vi "Part 2.vi"(11 "Input":string) -> (3 "Output":i64)   [LabVIEW 2021]
uses:
  d8bb4194-d316-453b-bd2f-f561d20e04f1.vi
  <userlib>/_OpenG.lib/string/string.llb/Convert EOLs (String)__ogtk.vi
  <vilib>/Comparison/Less/Less Functor/Less Functor.lvclass
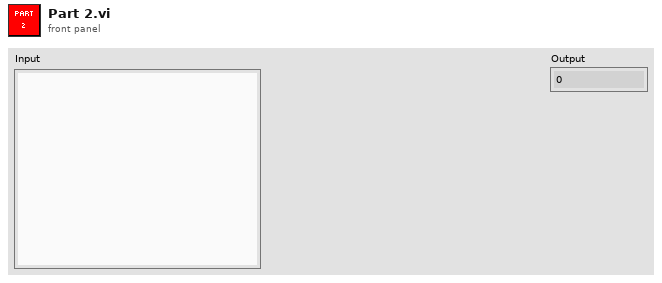
[diagram p1: front panel]
types:
  T1 = cluster{"Type":enum16{"High card", "One pair", "Two pair", "Three of a kind", "Full house", "Four of a kind", "Five of a kind"}, "Hand":string, "Bid":i64}
  T2 = enum16{"High card", "One pair", "Two pair", "Three of a kind", "Full house", "Four of a kind", "Five of a kind"}
  T3 = cluster{"Type":enum16{"High card", "One pair", "Two pair", "Three of a kind", "Full house", "Four of a kind", "Five of a kind"}, "Hand":string, "Bid":i64}[]
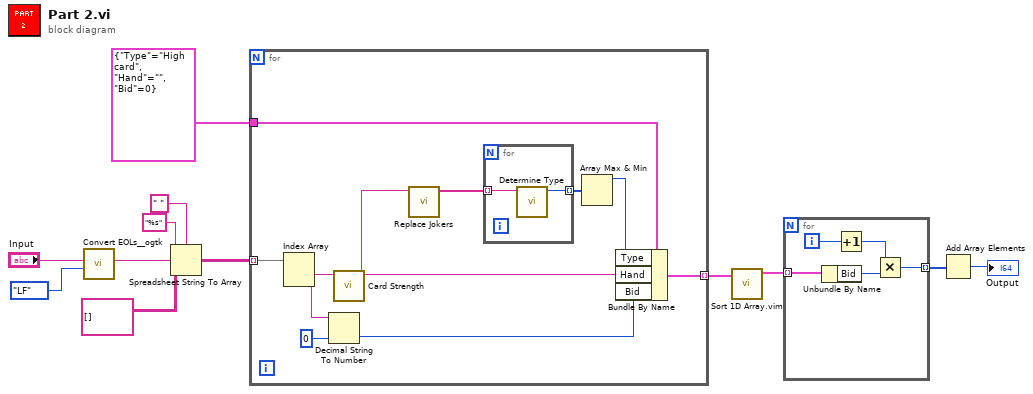
[diagram p0: block diagram]
diagram:
  n1 = call-poly <userlib>:"Convert EOLs__ogtk.vi"("Convert to:"=enum16{"CR", "LF", "CRLF"}."LF", "String in"="Input") -> ("String out"=w8:string)  [unwired: 9 in]
  n2 = Spreadsheet String To Array(delimiter (Tab)=" ", format string="%s", spreadsheet string=w8, array type (2D Dbl)=string[][] []) -> (array=w6:string[][])
  n3 = for {
    tunnel: w6 -> [w23] mode=indexing
    tunnel: T1 {"Type"=enum."High card", "Hand"="", "Bid"=0} ("output cluster") -> [w19]
    tunnel: [w20] -> w5 mode=indexing
    n4 = Index Array(array=w23) -> (element #1=w17:string, element #2=w22:string)  [unwired: 2 in]
    n5 = Decimal String To Number(string=w22, default (0L)=i64 0) -> (number=w18:i64)  [unwired: 1 in, 1 out]
    n6 = call "Card Strength.vi"("Hand In"=w17) -> ("Hand Out"=w15:string)  [unwired: 10 in]
    n7 = call "Replace Jokers.vi"("Hand"=w15) -> ("Possible Hands"=w13:string[])  [unwired: 10 in]
    n8 = for {
      tunnel: [w25] -> w16 mode=indexing
      tunnel: w13 -> [w24] mode=indexing
      n9 = call "Determine Type.vi"("Hand"=w24) -> ("Type"=w25:T2)  [unwired: 10 in]
    }
    n10 = Array Max & Min(array=w16) -> (max value=w14:T2)  [unwired: 3 out]
    n11 = Bundle By Name(cluster=w19, "Type"=w14, "Hand"=w15, "Bid"=w18) -> (w20:T1)
  }
  n12 = call "Sort 1D Array.vim"("unsorted array"=w5) -> ("sorted array"=w4:T3)  [unwired: 10 in]
  n13 = for {
    tunnel: w4 -> [w30] mode=indexing
    tunnel: [w26] -> w2 mode=indexing
    i -> [w29]
    n14 = Unbundle By Name(w30) -> ("Bid"=w28:i64)
    n15 = Increment(x=w29) -> (x+1=w27:i32)
    n16 = Multiply(x=w27, y=w28) -> (x*y=w26:i64)
  }
  n17 = Add Array Elements(numeric array=w2) -> (sum=→"Output":i64)
